vi "Configure.vi"(8 "error in (no error)":errorcluster, 9 "ActorMeter Enqueuer":refnum<class "Message Enqueuer.lvclass">, 10 "Name":string, 11 "Viewable Actor in":refnum<class "Viewable Actor.lvclass">) -> (0 "error out":errorcluster, 3 "Viewable Actor out":refnum<class "Viewable Actor.lvclass">)   [LabVIEW 2014, in "Viewable Actor.lvlib" / "Viewable Actor.lvclass"]
uses:
  Viewable Actor.lvclass
  <vilib>/ActorFramework/Message Enqueuer/Message Enqueuer.lvclass
  Viewable Actor.lvclass/Viewable Actor.ctl
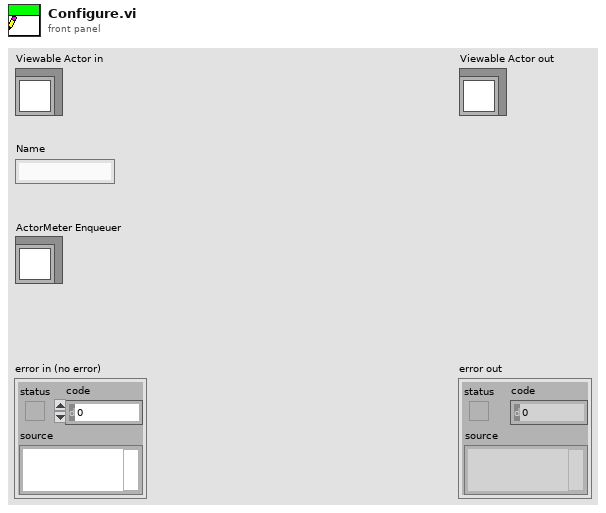
[diagram p1: front panel]
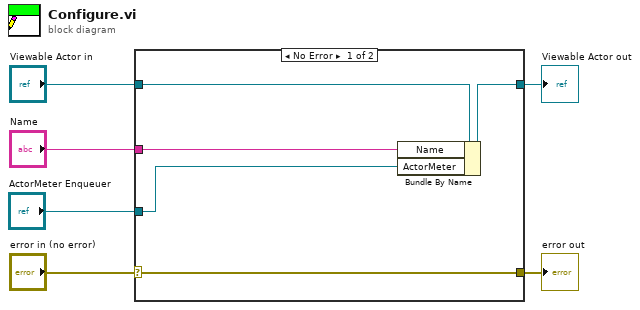
[diagram p0: block diagram]
diagram:
  n1 = case shown="No Error" "error in (no error)" {
    selector: "error in (no error)" -> [w11 w12]
    tunnel: [w11 w12] -> w5
    tunnel: [w9 w13] -> w3
    tunnel: "Viewable Actor in" -> [w10 w13]
    tunnel: "Name" -> [w8 _]
    tunnel: "ActorMeter Enqueuer" -> [w7 _]
    frame No Error {
      n2 = Bundle By Name(cluster=w10, "Name"=w8, "ActorMeter"=w7) -> (w9:refnum<class "Viewable Actor.lvclass">)
    }
    frame Error {
    }
  }
  "error out" <- w5
  "Viewable Actor out" <- w3
